vi "Enable Disable SLSC.vi"(8 "error in (no error)":errorcluster, 11 "Node Ptr":u64 format="%.0x") -> (0 "error out":errorcluster)   [LabVIEW 2014, in "SLSC configuration System Explorer.lvlib"]
uses:
  SLSC configuration System Explorer.lvlib
  Shared/Constants.vi
  <vilib>/NI Veristand/Custom Device API/Custom Device API.lvlib
  Shared/SLSC configuration Shared.lvlib
panel:
  in  "Tag":string
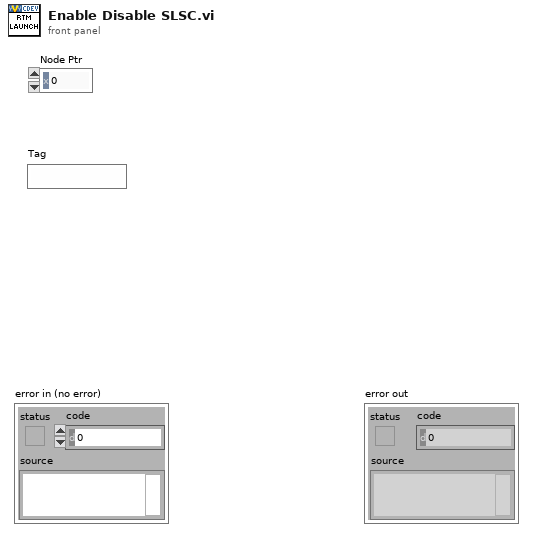
[diagram p1: front panel]
types:
  T1 = typedef "Custom Device API.lvlib/Custom Device Item Ref.ctl" = u64
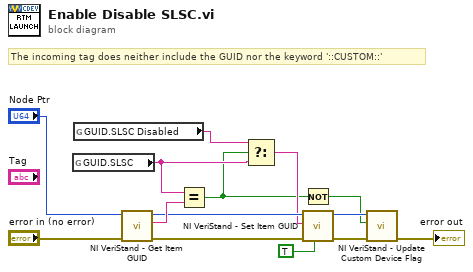
[diagram p0: block diagram]
diagram:
  # "The incoming tag does neither include the GUID nor the keyword '::CUSTOM::'"
  n1 = global read "Constants.vi" "GUID.SLSC"() -> (w10:string)
  n2 = global read "Constants.vi" "GUID.SLSC Disabled"() -> (w11:string)
  n3 = call <vilib>:"NI VeriStand - Get Item GUID.vi"("error in (no error)"="error in (no error)", "Item Ref in"="Node Ptr") -> ("error out"=w9:errorcluster, "GUID"=w12:string, "Item Ref out"=w8:T1)  [unwired: 7 in]
  n4 = Equal?(x=w10, y=w12) -> (x = y?=w3:bool)
  n5 = Select(t=w11, s=w3, f=w10) -> (s? t:f=w6:string)
  n6 = Not(x=w3) -> (.not. x?=w2:bool)
  n7 = call <vilib>:"NI VeriStand - Set Item GUID.vi"("Refresh System Explorer Tree? (F)"=TRUE, "error in (no error)"=w9, "GUID"=w6, "Item Ref in"=w8) -> ("error out"=w5:errorcluster, "Item Ref out"=w4:T1)  [unwired: 6 in]
  n8 = call <vilib>:"NI VeriStand - Update Custom Device Flag.vi"("error in (no error)"=w5, "Is Custom Device Active?"=w2, "Device Ref in"=w4) -> ("error out"=→"error out":errorcluster)  [unwired: 7 in, 1 out]
